vi "RunningAverage-GetGroupData.vi"(8 "Error in":errorcluster, 9 "Enable Array":bool[](array[boolean]), 11 "Device Ref in":T1 format="%.0x") -> (0 "Error out":errorcluster, 2 "Group Data Array":T2(array[cluster]) {"VS Refs" format="%.0x"}, 3 "Device Ref out":T1=18446744073709551615 format="%.0x")   [LabVIEW 2015, in "Waveform-Processing-Custom-Device Shared.lvlib" / "Running Average.lvlib"]
uses:
  Running Average.lvlib
  <vilib>/NI Veristand/Custom Device API/Custom Device Item Ref.ctl
  Constants.vi
  <vilib>/NI Veristand/Custom Device API/Get Item Property (Dependent Node Pointer).vi
  <vilib>/NI Veristand/Custom Device Tools/Custom Device Utility Library/NI VeriStand - Search for Item by GUID.vi
  System Explorer/Waveform-Processing-Custom-Device System Explorer.lvlib
  <vilib>/NI VeriStand/Custom Device API/Custom Device API.lvlib
  Waveform-Processing-Custom-Device Shared.lvlib
  <vilib>/NI Veristand/Custom Device Tools/Custom Device Utility Library/Custom Device Utility Library.lvlib
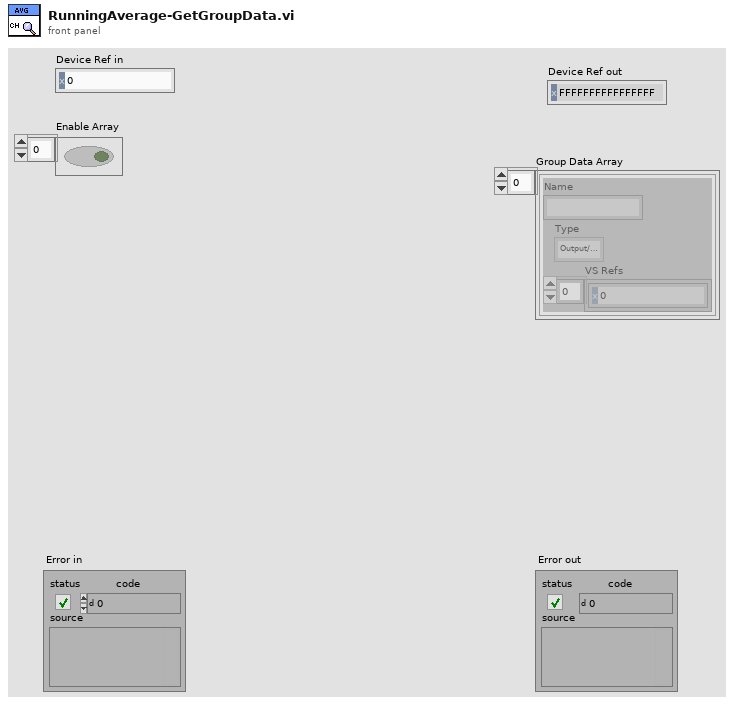
[diagram p1: front panel]
types:
  T1 = typedef "Custom Device API.lvlib/Custom Device Item Ref.ctl" = u64
  T2 = cluster{"Name":string, "Type":enum16{"Output/Write", "Input/Read", "Input/ReadWrite"}, "VS Refs":T1[]}[]
  T3 = enum16{"Output/Write", "Input/Read", "Input/ReadWrite"}
  T4 = cluster{"Name":string, "Type":enum16{"Output/Write", "Input/Read", "Input/ReadWrite"}, "VS Refs":T1[]}
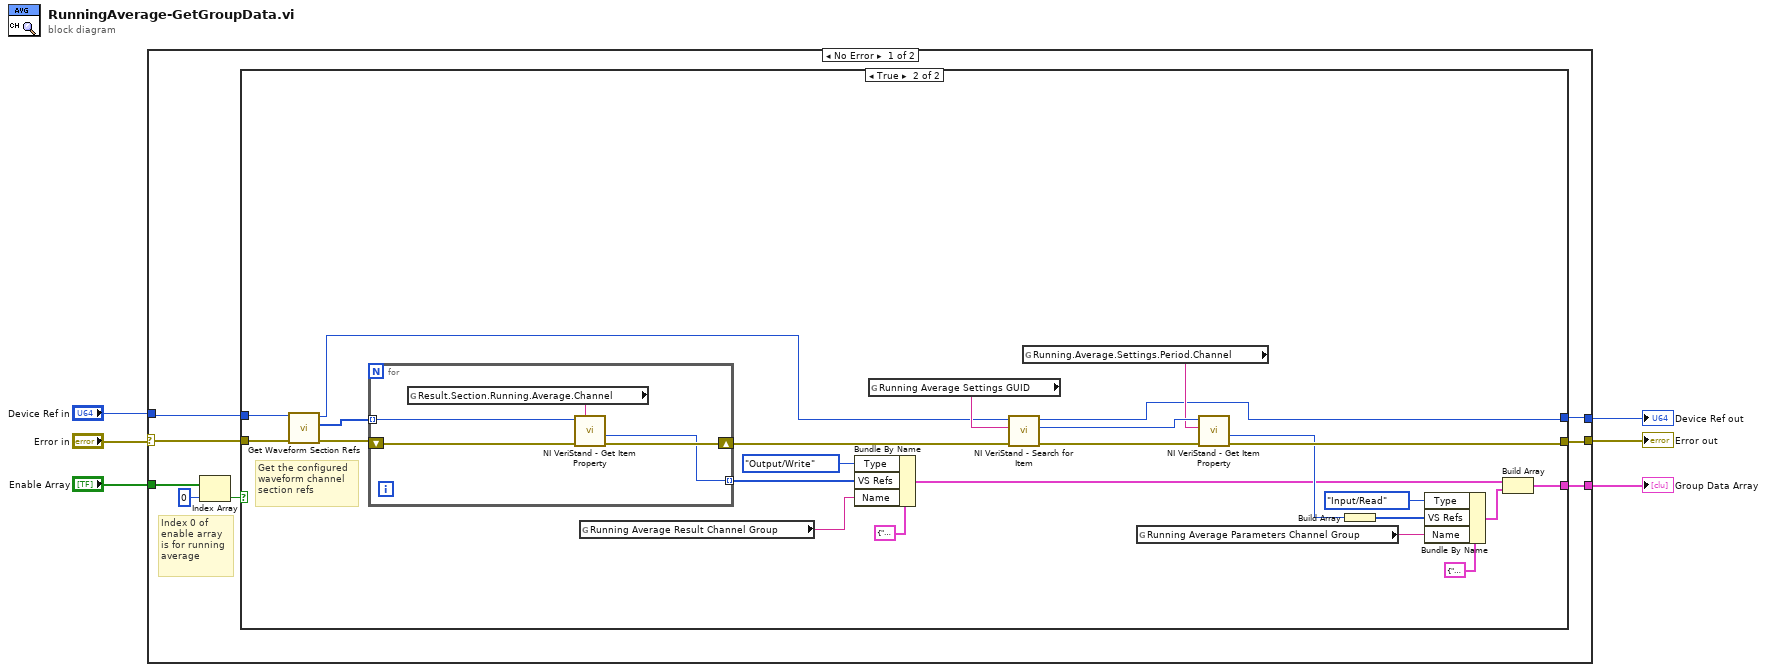
[diagram p0: block diagram]
diagram:
  n1 = case shown="No Error" "Error in" {
    selector: "Error in" -> [w14 w47]
    tunnel: [w12 w47] -> w5
    tunnel: "Device Ref in" -> [w13 w46]
    tunnel: [w11 w46] -> w3
    tunnel: [w10 _] -> w2
    tunnel: "Enable Array" -> [w8 _]
    frame No Error {
      # "Index 0 of\nenable array\nis for running\naverage"
      n2 = Index Array(array=w8, index=0) -> (element=w9:bool)
      n3 = case shown="True" w9 {
        tunnel: w14 -> [w16 w40]
        tunnel: w13 -> [w15 w38]
        tunnel: [w16 w31] -> w12
        tunnel: [w15 w30] -> w11
        tunnel: [_ w17] -> w10
        frame False {
        }
        frame True {
          # "Get the configured\nwaveform channel\nsection refs"
          n4 = call "Get Waveform Section Refs.vi"("Error in"=w40, "Device Ref in"=w38) -> ("Error out"=w39:errorcluster, "Result Section Refs"=w37:T1[], "Device Ref out"=w28:T1)  [unwired: 7 in]
          n5 = for {
            tunnel: w37 -> [w41] mode=indexing
            shift-right: [w43] -> w36
            shift-left: w39 -> [w45]
            tunnel: [w42] -> w29 mode=indexing
            n6 = global read "Constants.vi" "Result.Section.Running.Average.Channel"() -> (w44:string)
            n7 = call-poly <vilib>:"NI VeriStand - Get Item Property.vi"("error in (no error)"=w45, "Property Name"=w44, "Item Ref in"=w41) -> ("error out"=w43:errorcluster, "Dependent Node Ref"=w42:T1)  [unwired: 5 in, 2 out]
          }
          n8 = global read "Constants.vi" "Running Average Result Channel Group"() -> (w27:string)
          n9 = Bundle By Name(cluster=T4 {"Name"="", "Type"=enum."Output/Write", "VS Refs"=[]} ("Group"), "Type"=T3."Output/Write", "VS Refs"=w29, "Name"=w27) -> (w19:T4)
          n10 = global read "Constants.vi" "Running Average Settings GUID"() -> (w35:string)
          n11 = call-poly <vilib>:"NI VeriStand - Search for Item.vi"("error in"=w36, "Item GUID"=w35, "Section Ref in"=w28) -> ("error out"=w34:errorcluster, "Item Ref"=w33:T1, "Section Ref out"=w30:T1)  [unwired: 5 in, 1 out]
          n12 = global read "Constants.vi" "Running.Average.Settings.Period.Channel"() -> (w32:string)
          n13 = global read "Constants.vi" "Running Average Parameters Channel Group"() -> (w22:string)
          n14 = call-poly <vilib>:"NI VeriStand - Get Item Property.vi"("error in (no error)"=w34, "Property Name"=w32, "Item Ref in"=w33) -> ("error out"=w31:errorcluster, "Dependent Node Ref"=w21:T1)  [unwired: 5 in, 2 out]
          n15 = Build Array(w21) -> (w20:T1[])
          n16 = Bundle By Name(cluster=T4 {"Name"="", "Type"=enum."Output/Write", "VS Refs"=[]} ("Group"), "Type"=T3."Input/Read", "VS Refs"=w20, "Name"=w22) -> (w18:T4)
          n17 = Build Array(w19, w18) -> (w17:T2)
        }
      }
    }
    frame Error {
    }
  }
  "Error out" <- w5
  "Device Ref out" <- w3
  "Group Data Array" <- w2
